vi "Get SLSC Modules By GUID.vi"(8 "error in (no error)":errorcluster, 10 "GUID":string, 11 "SLSC Chassis":u64) -> (0 "error out":errorcluster, 1 "Found":bool, 2 "SLSC Modules":u64[](array[numeric]), 3 "SLSC Chassis out":u64)   [LabVIEW 2020, in "VeriStand SLSC Scripting.lvlib"]
uses:
  VeriStand SLSC Scripting.lvlib
  NationalInstruments.VeriStand.SystemDefinitionAPI
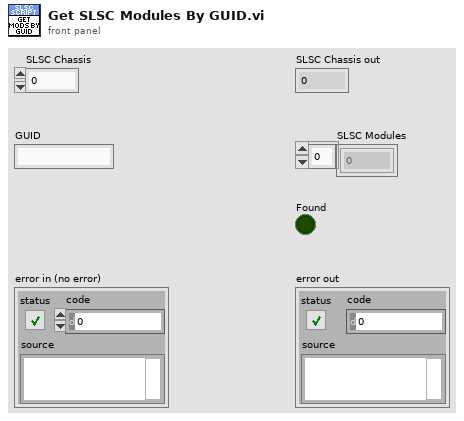
[diagram p1: front panel]
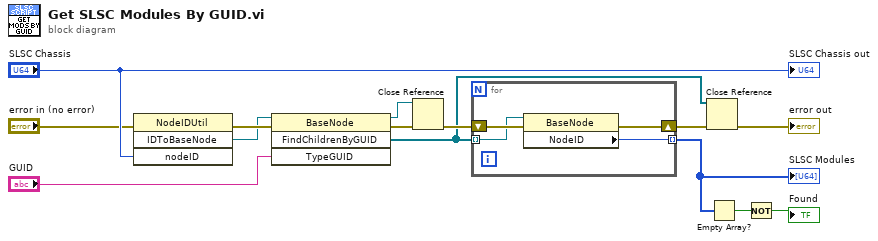
[diagram p0: block diagram]
diagram:
  n1 = invoke class="NodeIDUtil" method="IDToBaseNode"(error in="error in (no error)", "nodeID"="SLSC Chassis") -> (error out=w9:errorcluster, "IDToBaseNode"=w8:refnum<k24>)  [unwired: 2 in, 2 out]
  n2 = invoke class="BaseNode" method="FindChildrenByGUID"(reference=w8, error in=w9, "TypeGUID"="GUID") -> (reference out=w5:refnum<k24>, error out=w6:errorcluster, "FindChildrenByGUID"=w4:refnum<k24>[])  [unwired: 1 in, 1 out]
  n3 = Close Reference(reference=w5, error in (no error)=w6) -> (error out=w12:errorcluster)
  n4 = for {
    shift-right: [w17] -> w11
    shift-left: w12 -> [w18]
    tunnel: w4 -> [w16] mode=indexing
    tunnel: [w15] -> w3 mode=indexing
    n5 = property class="BaseNode"(reference=w16, error in=w18) -> (error out=w17:errorcluster, "NodeID"=w15:u64)  [unwired: 1 out]
  }
  "SLSC Modules" <- w3
  n6 = Close Reference(reference=w4, error in (no error)=w11) -> (error out=→"error out":errorcluster)
  n7 = Empty Array?(array=w3) -> (empty?=w2:bool)
  n8 = Not(x=w2) -> (.not. x?=→"Found":bool)
  "SLSC Chassis out" <- "SLSC Chassis"
